vi "trig.vi"(2 "s":bool, 3 "c":bool, 4 "d":bool, 5 "r":bool) -> (0 "not q":bool, 1 "q":bool)   [LabVIEW 2012]
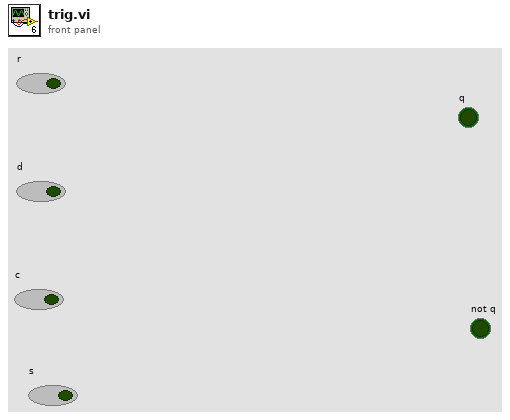
[diagram p1: front panel]
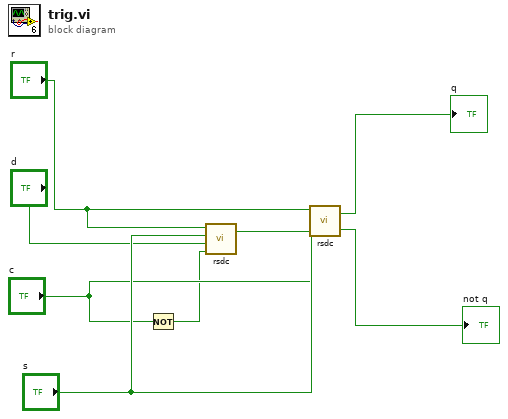
[diagram p0: block diagram]
diagram:
  n1 = Not(x="c") -> (.not. x?=w3:bool)
  n2 = call "rsdc.vi"("c"=w3, "d"="d", "s"="s", "r"="r") -> ("q"=w5:bool)  [unwired: 1 out]
  n3 = call "rsdc.vi"("c"="c", "d"=w5, "s"="s", "r"="r") -> ("not q"=→"not q":bool, "q"=→"q":bool)
